vi "RMPS Globals.vi"() -> ()   [LabVIEW 2018]
doc: "Author: Scott Hannahs <sth@magnet.fsu.edu>\nCopyright 2018 Florida State University, All rights reserved."
panel:
  in  "# Cycles To Activate":u32=5
  in  "Actual Cycle Time":dbl format="%.6f"
  in  "Recording Interval":dbl=2.0 format="%.1f"
  out "RMPS Data Queue":refnum<queue>
  in  "Activation Current":dbl=1.0 format="%.1f"
  in  "# Non-coil Channels":u32=11
  in  "Max Board Acq Rate":dbl=95000.0
  in  "Cycle Freq":dbl=30.0 format="%.3f"
  out "DAQ Buffer Size":u32
  in  "Posttrigger Sec of Data":dbl=10.0 format="%.2f"
  in  "Pretrigger sec of data":dbl=30.0 format="%.2f"
  in  "Magnet Data":dbl[](array[numeric]) format="%.3f"
  in  "# Scans to read":i32
  out "Seconds/Scan":dbl format="%^.4e"
  out "Digital  IO Task":refnum<k21>
  out "Analog taskID":refnum<k21>
  out "# Coils":u32
  # "Tin"
  # "Tout"
  # "Pin"
  # "Pout"
  # "Current"
  # "WDTimer"
  # "PSenb"
  # "Cell Fault"
  # "WDTrip"
  # "BT Trip"
  # "BT Volts"
  # "Va"
  # "Vb"
  # "Vc"
  # "Vd"
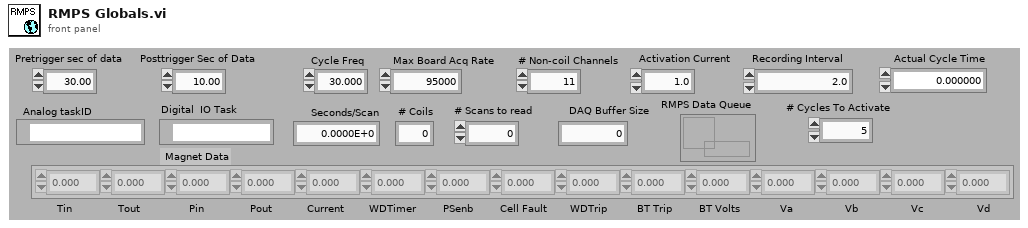
[diagram p1: front panel]
diagram:
